vi "Random Samples.vi"(9 "# Picks":i32, 11 "Input Array":dbl[](array[numeric])) -> (2 "Samples":dbl[](array[numeric]))   [LabVIEW 2013]
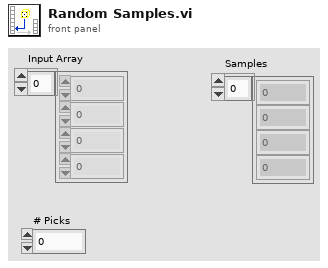
[diagram p1: front panel]
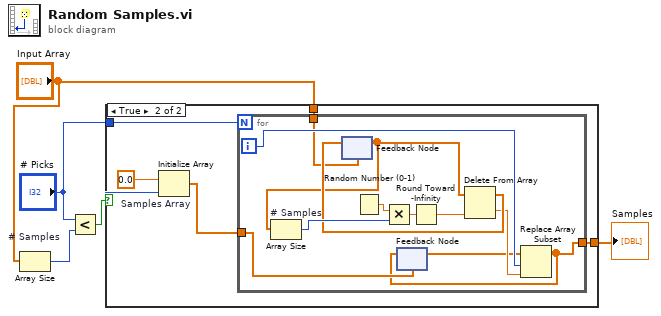
[diagram p0: block diagram]
diagram:
  n1 = Array Size "# Samples"(array="Input Array") -> (size(s)=w3:i32)
  n2 = Less?(x="# Picks", y=w3) -> (x < y?=w1:bool)
  n3 = case shown="True" w1 {
    tunnel: "# Picks" -> [_ w10]
    tunnel: [w6 w8] -> w5
    tunnel: "Input Array" -> [w6 w7]
    frame False {
    }
    frame True {
      n4 = Initialize Array "Samples Array"(0.0, w10) -> (w9:dbl[])
      n5 = for {
        N: w10 -> [_]
        tunnel: w7 -> [w13]
        tunnel: w9 -> [w15]
        tunnel: [w14] -> w8
        i -> [w18]
        n6 = feedback #1(w13) -> (w12:dbl[])
        n7 = Array Size "# Samples"(array=w12) -> (size(s)=w20:i32)
        n8 = Random Number (0-1)() -> (number: 0 to 1=w23:dbl)
        n9 = Multiply(x=w23, y=w20) -> (x*y=w22:dbl)
        n10 = feedback #2(w15) -> (w16:dbl[])
        n11 = Round Toward -Infinity(1:w22) -> (0:w21:dbl)
        n12 = Delete From Array(array=w12, index=w21) -> (deleted portion=w17:dbl, array with subset deleted=w19:dbl[])  [unwired: 1 in]
        n13 = feedback-in #1(w19) -> ()
        n14 = Replace Array Subset(array=w16, new element=w17, index=w18) -> (w14:dbl[])
        n15 = feedback-in #2(w14) -> ()
      }
    }
  }
  "Samples" <- w5
